vi "USB - Wait.vi"(8 "error in":errorcluster, 11 "VISA Resource Name In":refnum<visa-resource-name>) -> (0 "error out":errorcluster, 3 "VISA Resource Name Out":refnum<visa-resource-name>)   [LabVIEW 2021]
doc: "Create a delay, to allow the device enough time to receive the command.\n\nThe wait time is defined by \"Constant - Wait Time (ms).vi\""
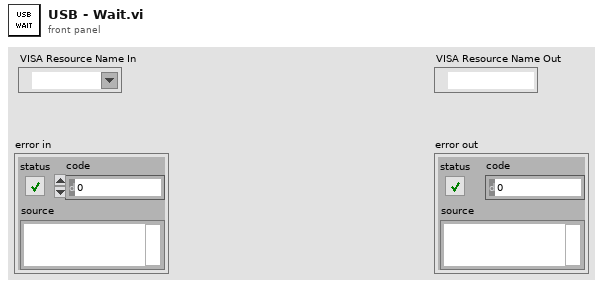
[diagram p1: front panel]
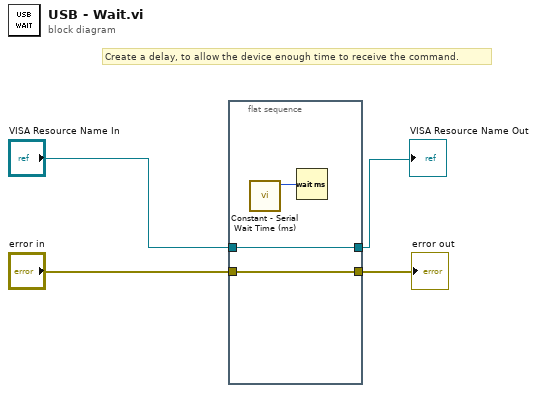
[diagram p0: block diagram]
diagram:
  # "Create a delay, to allow the device enough time to receive the command."
  n1 = flat-sequence {
    tunnel: "error in" -> [w7]
    tunnel: [w7] -> w3
    tunnel: "VISA Resource Name In" -> [w6]
    tunnel: [w6] -> w4
    frame #0 {
      n2 = call "Constant - Serial Wait Time (ms).vi"() -> ("milliseconds to wait"=w5:u32)  [unwired: 11 in]
      n3 = Wait (ms)(milliseconds to wait=w5) -> ()  [unwired: 1 out]
    }
  }
  "error out" <- w3
  "VISA Resource Name Out" <- w4
